vi "Simply Polymorphic (numeric).vi"(10 "Numeric Control":dbl) -> (2 "Numeric Indicator":dbl)   [LabVIEW 2011]
doc: "Instance VI used in a Polymorphic demonstration. Students can use it as well when getting started with polymorphic VIs.\n\nAAL 9/09"
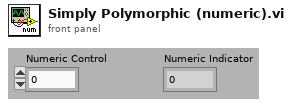
[diagram p1: front panel]
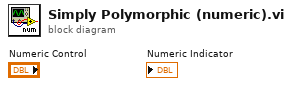
[diagram p0: block diagram]
diagram:
